vi "convert_two_complementary.vi"(4 "number in":i16=28) -> (1 "complementary out":i16)   [LabVIEW 2010]
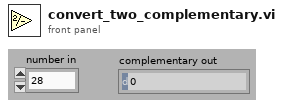
[diagram p1: front panel]
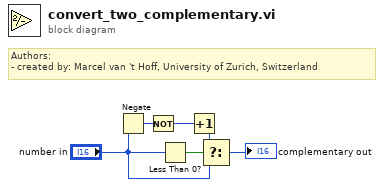
[diagram p0: block diagram]
diagram:
  # "Authors: \n- created by: Marcel van 't Hoff, University of Zurich, Switzerland"
  n1 = Negate(x="number in") -> (-x=w2:i16)
  n2 = Not(x=w2) -> (.not. x?=w1:i16)
  n3 = Less Than 0?(x="number in") -> (x < 0?=w3:bool)
  n4 = Increment(x=w1) -> (x+1=w5:i16)
  n5 = Select(t=w5, s=w3, f="number in") -> (s? t:f=→"complementary out":i16)
